vi "STSatZ.vi"() -> ()   [LabVIEW 2014]
uses:
  <userlib>/Nanonis Prog Interface V5/Nanonis Prog Interface.lvlib
panel:
  in  "z step":dbl format="%#_6p"
  in  "z range":dbl format="%#_6p"
  out "points":i32
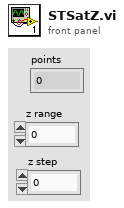
[diagram p1: front panel]
types:
  T1 = cluster{"center X (m)":sgl, "center Y (m)":sgl, "width (m)":sgl, "height (m)":sgl, "angle (deg)":sgl}
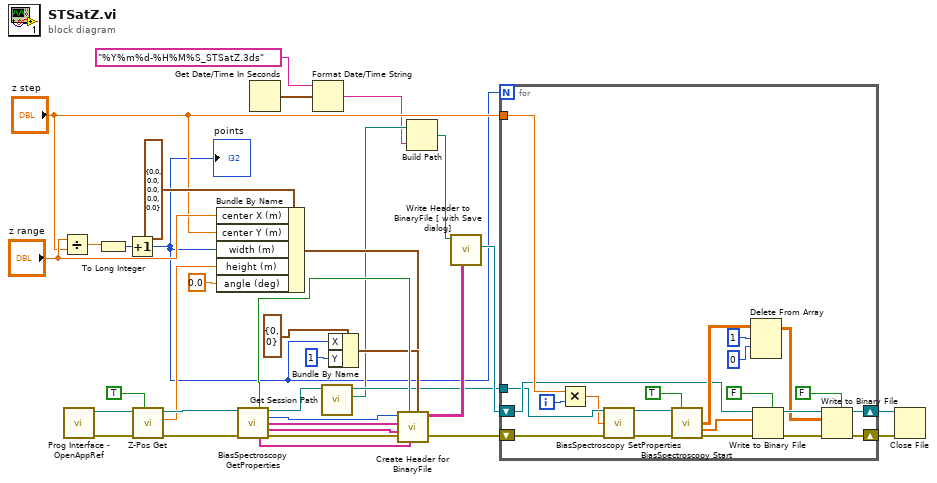
[diagram p0: block diagram]
diagram:
  n1 = Divide(x="z range", y="z step") -> (x/y=w33:dbl)
  n2 = call <userlib>:"Prog Interface - OpenAppRef.vi"() -> ("Error out"=w14:errorcluster, "Application reference"=w15:refnum<vi>)  [unwired: 6 in]
  n3 = To Long Integer(number=w33) -> (32bit integer=w16:i32)
  n4 = Increment(x=w16) -> (x+1=w1:i32)
  "points" <- w1
  n5 = call <userlib>:"Z-Pos Get.vi"("Wait for newest data (F=False)"=TRUE, "error in (no error)"=w14, "Application ref in"=w15) -> ("error out"=w12:errorcluster, "Z position (m)"=w10:sgl, "Application ref out"=w13:refnum<vi>)  [unwired: 6 in]
  n6 = Bundle By Name(cluster=T1 {"center X (m)"=0.0, "center Y (m)"=0.0, "width (m)"=0.0, "height (m)"=0.0, "angle (deg)"=0.0} ("Grid param"), "center X (m)"="z range", "center Y (m)"="z step", "width (m)"=w1, "height (m)"=w10, "angle (deg)"=sgl 0.0) -> (w19:T1)
  n7 = call <userlib>:"BiasSpectroscopy GetProperties.vi"("Application ref in"=w13, "Error in (no error)"=w12) -> ("Backward sweep"=w28:bool, "Application ref out"=w8:refnum<vi>, "Number of points"=w29:i32, "Channels"=w31:string[], "Parameters"=w32:string[], "Fixed parameters"=w30:string[], "Error out"=w11:errorcluster)  [unwired: 5 in, 2 out]
  n8 = Get Date/Time In Seconds() -> (seconds since 1Jan1904=w4:timestamp)
  n9 = Format Date/Time String(time format string (%c)="%Y%m%d-%H%M%S_STSatZ.3ds", seconds (now)=w4) -> (date/time string=w2:string)  [unwired: 1 in]
  n10 = call <userlib>:"Get Session Path.vi"("Application ref in"=w8) -> ("Session path"=w6:path, "Application ref out"=w7:refnum<vi>)  [unwired: 8 in, 1 out]
  n11 = Bundle By Name(cluster=cluster{"X":i32, "Y":i32} {"X"=0, "Y"=0} ("Grid points"), "X"=w1, "Y"=1) -> (w22:cluster{"X":i32, "Y":i32})
  n12 = call <userlib>:"Create Header for BinaryFile.vi"("Grid points"=w22, "Grid param"=w19, "Fixed parameters"=w30, "Backward sweep"=w28, "Parameters"=w32, "Channels"=w31, "Points per sweep"=w29) -> ("Header (fixed attributes)"=w27:string[][])  [unwired: 4 in]
  n13 = Build Path(base path=w6, name or relative path=w2) -> (appended path=w5:path)
  n14 = call <userlib>:"Write Header to BinaryFile [ with Save dialog].vi"("Fixed Attributes"=w27, "Filename"=w5) -> ("File ref"=w26:refnum<file>)  [unwired: 6 in, 3 out]
  n15 = for {
    N: w1 -> [_]
    tunnel: "z step" -> [w54]
    tunnel: w7 -> [w39]
    shift-right: [w42] -> w25
    shift-left: w26 -> [w40]
    shift-right: [w41] -> w24
    shift-left: w11 -> [w37]
    i -> [w55]
    n16 = Multiply(x=w54, y=w55) -> (x*y=w35:dbl)
    n17 = call <userlib>:"BiasSpectroscopy SetProperties.vi"("Application ref in"=w39, "Z offset (m) (NaN=no change)"=w35, "Error in (no error)"=w37) -> ("Application ref out"=w38:refnum<vi>, "Error out"=w36:errorcluster)  [unwired: 11 in]
    n18 = call <userlib>:"BiasSpectroscopy Start.vi"("Application ref in"=w38, "Get data (F)"=TRUE, "Error in (no error)"=w36) -> ("Data"=w45:sgl[][], "Parameters"=w43:sgl[], "Error out"=w44:errorcluster)  [unwired: 8 in, 2 out]
    n19 = Delete From Array(array=w45, length=1, index (row)=0 ("index")) -> (array with subset deleted=w51:sgl[][])  [unwired: 1 in, 1 out]
    n20 = Write to Binary File(file (use dialog)=w40, data=w43, error in=w44, 5:FALSE ("prepend array or string size? (T)")) -> (refnum out=w52:refnum<file>, error out=w46:errorcluster)  [unwired: 2 in, 1 out]
    n21 = Write to Binary File(file (use dialog)=w52, data=w51, error in=w46, 5:FALSE ("prepend array or string size? (T)")) -> (refnum out=w42:refnum<file>, error out=w41:errorcluster)  [unwired: 2 in, 1 out]
  }
  n22 = Close File(refnum=w25, error in=w24) -> ()  [unwired: 2 out]
